vi "HOST_TASCA.vi"() -> ()   [LabVIEW 2013]
uses:
  <vilib>/FPGAPlugInAG/cRIO-9075/niLvFpga_Open_cRIO-9075.vi
  <vilib>/rvi/interface/common/dynamic/niFpgaDynamicAddResources.vi
  <vilib>/rvi/interface/common/niFpgaWaitOnOcc.vi
  <vilib>/Utility/error.llb/Error Cluster From Error Code.vi
  <vilib>/rvi/errors/niLvFpgaAdjustHostInterfaceError.vi
  <vilib>/FPGAPlugInAG/Dynamic/niLvFpga_Run_Dynamic.vi
  <vilib>/RVI Host/nirviSupport.llb/nirviErrorClusterFromErrorCode.vi
  <vilib>/FPGAPlugInAG/Dynamic/niLvFpga_Close_Dynamic.vi
  <vilib>/rvi/interface/nirviOpenFPGA/nirviOpenFPGA.xnode
  Users/loqufrj/Desktop/Malena_FPGA/FPGA Bitfiles/ProjetoTasca_FPGATarget_ProjetoTASCA_6hheV-3e9N0.lvbitx
  Users/loqufrj/Desktop/Malena_FPGA/ProjetoTASCA.vi
  <vilib>/rvi/interface/nirviReadWriteControl/nirviReadWriteControl.xnode
  <vilib>/rvi/interface/nirviMethod/nirviMethod.xnode
  <vilib>/rvi/interface/nirviCloseFPGA/nirviCloseFPGA.xnode
  <vilib>/rvi/interface/Simulation/niFpgaSimulationCallBeginRW.vi
  NiFpgaLv.dll
  <vilib>/rvi/interface/nirviMethod/StockFPGA_InlinedMethodWaitForSingleIRQ.vi
  <vilib>/FPGAPlugInAG/Dynamic/niLvFpga_WaitOnIrq_Dynamic.vi
panel:
  out "Coincidences":u32
  out "Count 1":u32
  out "Loop execution time":u32=4
  out "0 Chart":u32(graph)
  in  "stop":bool
  out "Count 0":u32
  in  "Measurement Time (s)":sgl=1.0
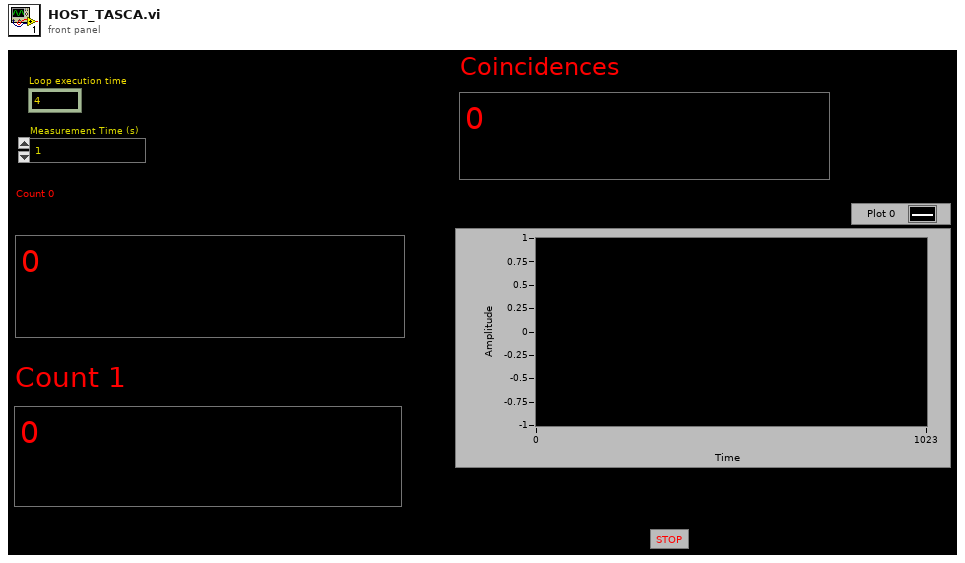
[diagram p1: front panel]
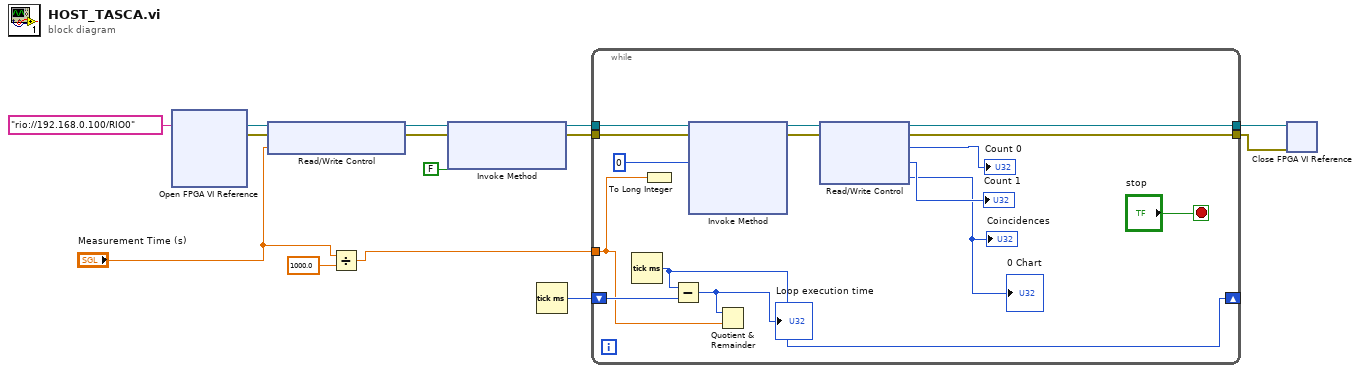
[diagram p0: block diagram]
diagram:
  n1 = xnode "Open FPGA VI Reference"("resource name"=tag "rio://192.168.0.100/RIO0") -> ("FPGA VI Reference Out"=w14:refnum<k20>, "error out"=w13:errorcluster)  [unwired: 1 in]
  n2 = xnode "Read/Write Control"("FPGA VI Reference In"=w14, "error in"=w13, "Measurement Time (s)"="Measurement Time (s)") -> ("FPGA VI Reference Out"=w8:refnum<k20>, "error out"=w7:errorcluster)
  n3 = Divide(x="Measurement Time (s)", y=sgl 1000.0) -> (x/y=w2:sgl)
  n4 = xnode "Invoke Method"("FPGA VI Reference In"=w8, "error in"=w7, "Wait Until Done (F)"=FALSE) -> ("FPGA VI Reference Out"=w6:refnum<k20>, "error out"=w5:errorcluster)
  n5 = Tick Count (ms)() -> (millisecond timer value=w1:u32)
  n6 = while {
    tunnel: [w27] -> w12
    tunnel: [w26] -> w11
    tunnel: w6 -> [w28]
    tunnel: w5 -> [w20]
    tunnel: w2 -> [w16]
    shift-right: [w23] -> _
    shift-left: w1 -> [w24]
    stop <- "stop" stop-if-true
    n7 = Tick Count (ms)() -> (millisecond timer value=w23:u32)
    n8 = To Long Integer(number=w16) -> ()  [unwired: 1 out]
    n9 = Subtract(x=w23, y=w24) -> (x-y=w25:u32)
    "Loop execution time" <- w25
    n10 = xnode "Invoke Method"("FPGA VI Reference In"=w28, "error in"=w20, "IRQ Number(s)"=0) -> ("FPGA VI Reference Out"=w21:refnum<k20>, "error out"=w19:errorcluster)  [unwired: 1 in, 2 out]
    n11 = Quotient & Remainder(x=w25, y=w16) -> ()  [unwired: 2 out]
    n12 = xnode "Read/Write Control"("FPGA VI Reference In"=w21, "error in"=w19) -> ("FPGA VI Reference Out"=w27:refnum<k20>, "error out"=w26:errorcluster, "Count 0"=→"Count 0":u32, "Count 1"=→"Count 1":u32, "Coincidences"=→"0 Chart" →"Coincidences":u32)
  }
  n13 = xnode "Close FPGA VI Reference"("FPGA VI Reference In"=w12, "error in"=w11) -> ()  [unwired: 1 out]
